vi "Anritsu VNA Read Measurement.vi"(4 "Trace":i8=1 min=1 max=99 step=1, 6 "Channel":i8=1 min=1 max=99 step=1, 7 "Anritsu VNA":T1, 8 "error in (no error)":errorcluster, 11 "VISA Resource Name":refnum<visa-resource-name>) -> (0 "error out":errorcluster, 1 "Parameter":T2={"Stimulus Port"=1, "Response Port"=1} {"Stimulus Port" min=1 step=1; "Response Port" min=1 step=1}, 3 "dup VISA Resource Name":refnum<visa-resource-name>)   [LabVIEW 2011]
doc: "This VI = the HP 8753B is used to read the meausurement format.\n\n0 log magnitude\n1 phase\n2 delay\n3 Smith chart\n4 polar\n5 linear magnitude\n6 standing wave ratio\n7 real\n8 imaginary"
uses:
  tests/S Parameter/TypeDefs/SP Parameter.ctl
  TypeDefs/Anritsu VNA Instrument Info.ctl
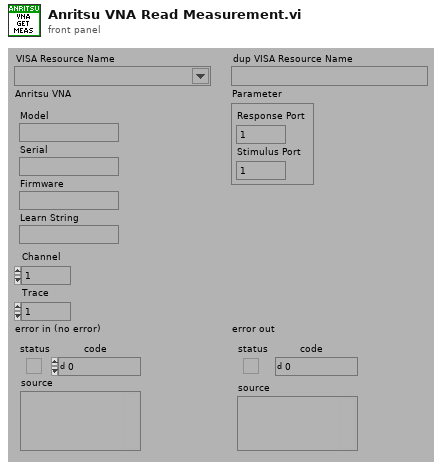
[diagram p1: front panel]
types:
  T1 = typedef "Anritsu VNA Instrument Info.ctl" = cluster{"Model":string, "Serial":string, "Firmware":string, "Learn String":string}
  T2 = typedef "SP Parameter.ctl" = cluster{"Stimulus Port":i8, "Response Port":i8}
  T3 = typedef "Anritsu VNA Model.ctl" = enum16{"Not Supported", "37XXXX", "MS20XXX", "MS462XX", "MS464XX"}
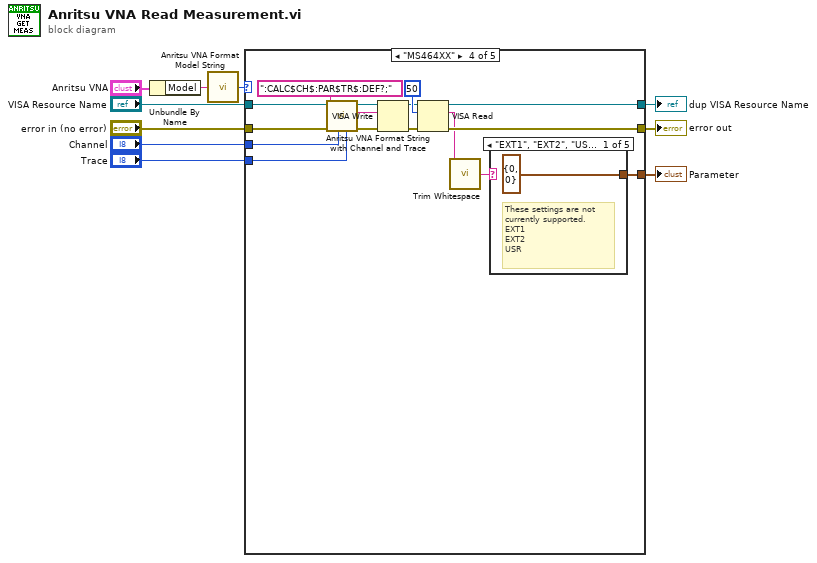
[diagram p0: block diagram]
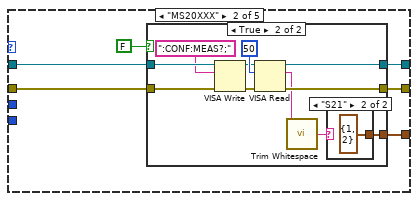
[diagram p3: hidden frame]
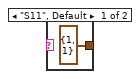
[diagram p5: hidden frame]
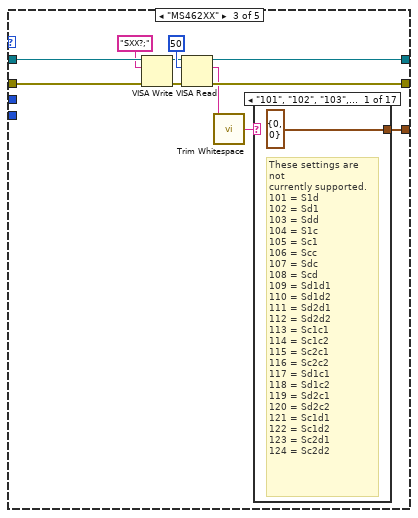
[diagram p6: hidden frame]
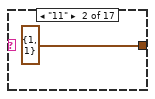
[diagram p7: hidden frame]
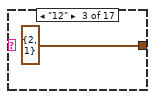
[diagram p8: hidden frame]
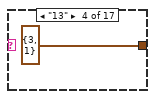
[diagram p9: hidden frame]
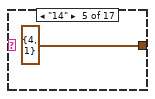
[diagram p10: hidden frame]
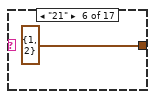
[diagram p11: hidden frame]
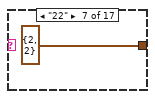
[diagram p12: hidden frame]
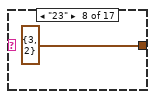
[diagram p13: hidden frame]
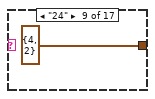
[diagram p14: hidden frame]
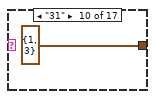
[diagram p15: hidden frame]
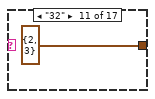
[diagram p16: hidden frame]
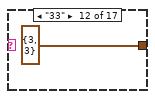
[diagram p17: hidden frame]
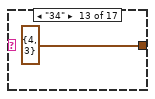
[diagram p18: hidden frame]
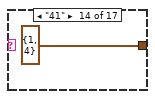
[diagram p19: hidden frame]
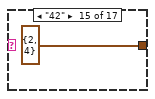
[diagram p20: hidden frame]
diagram:
  n1 = Unbundle By Name("Anritsu VNA") -> ("Model"=w4:string)
  n2 = call "Anritsu VNA Format Model String.vi"("Model"=w4) -> ("Model"=w3:T3)
  n3 = case shown="\"MS464XX\"" w3 {
    tunnel: "VISA Resource Name" -> [w11 w15 w41 w72 w88]
    tunnel: "error in (no error)" -> [w12 w18 w44 w75 w91]
    tunnel: [w12 w17 w43 w74 w90] -> w8
    tunnel: [_ w14 w40 w71 w87] -> w7
    tunnel: [w11 w16 w42 w73 w89] -> w6
    tunnel: "Channel" -> [_ _ _ w63 _]
    tunnel: "Trace" -> [_ _ _ w62 _]
    frame "Not Supported" {
    }
    frame "MS20XXX" {
      n4 = case shown="True" FALSE {
        tunnel: w18 -> [w19 w29]
        tunnel: [w19 w27] -> w17
        tunnel: [w20 w26] -> w16
        tunnel: w15 -> [w20 w25]
        tunnel: [_ w22] -> w14
        frame False {
        }
        frame True {
          n5 = VISA Write(VISA resource name=w25, write buffer=":CONF:MEAS?;", error in (no error)=w29) -> (VISA resource name out=w30:refnum<visa-resource-name>, error out=w28:errorcluster)  [unwired: 1 out]
          n6 = VISA Read(VISA resource name=w30, byte count=u32 50, error in (no error)=w28) -> (VISA resource name out=w26:refnum<visa-resource-name>, read buffer=w24:string, error out=w27:errorcluster)  [unwired: 1 out]
          n7 = call <vilib>:"Trim Whitespace.vi"("string"=w24) -> ("trimmed string"=w23:string)  [unwired: 1 in]
          n8 = case shown="\"S21\"" w23 {
            tunnel: [T2 {"Stimulus Port"=1, "Response Port"=1} ("Display Format") T2 {"Stimulus Port"=1, "Response Port"=2} ("Display Format")] -> w22
            frame "S11", Default {
            }
            frame "S21" {
            }
          }
        }
      }
    }
    frame "MS462XX" {
      n9 = VISA Write(VISA resource name=w41, write buffer="SXX?;", error in (no error)=w44) -> (VISA resource name out=w38:refnum<visa-resource-name>, error out=w37:errorcluster)  [unwired: 1 out]
      n10 = VISA Read(VISA resource name=w38, byte count=u32 50, error in (no error)=w37) -> (VISA resource name out=w42:refnum<visa-resource-name>, read buffer=w36:string, error out=w43:errorcluster)  [unwired: 1 out]
      n11 = call <vilib>:"Trim Whitespace.vi"("string"=w36) -> ("trimmed string"=w35:string)  [unwired: 1 in]
      n12 = case shown="\"101\", \"102\", \"103\", \"104\", \"105\", \"106\", \"107\", \"108\", \"109\", \"110\", \"111\", \"112\", \"113\", \"114\", \"115\", \"116\", \"117\", \"118\", \"119\", \"120\", \"121\", \"122\", \"123\", \"124\", Default" w35 {
        tunnel: [T2 {"Stimulus Port"=0, "Response Port"=0} ("Display Format") T2 {"Stimulus Port"=1, "Response Port"=1} ("Display Format") T2 {"Stimulus Port"=2, "Response Port"=1} ("Display Format") T2 {"Stimulus Port"=3, "Response Port"=1} ("Display Format") T2 {"Stimulus Port"=4, "Response Port"=1} ("Display Format") T2 {"Stimulus Port"=1, "Response Port"=2} ("Display Format") T2 {"Stimulus Port"=2, "Response Port"=2} ("Display Format") T2 {"Stimulus Port"=3, "Response Port"=2} ("Display Format") T2 {"Stimulus Port"=4, "Response Port"=2} ("Display Format") T2 {"Stimulus Port"=1, "Response Port"=3} ("Display Format") T2 {"Stimulus Port"=2, "Response Port"=3} ("Display Format") T2 {"Stimulus Port"=3, "Response Port"=3} ("Display Format") T2 {"Stimulus Port"=4, "Response Port"=3} ("Display Format") T2 {"Stimulus Port"=1, "Response Port"=4} ("Display Format") T2 {"Stimulus Port"=2, "Response Port"=4} ("Display Format") T2 {"Stimulus Port"=3, "Response Port"=4} ("Display Format") T2 {"Stimulus Port"=4, "Response Port"=4} ("Display Format")] -> w40
        frame "101", "102", "103", "104", "105", "106", "107", "108", "109", "110", "111", "112", "113", "114", "115", "116", "117", "118", "119", "120", "121", "122", "123", "124", Default {
          # "These settings are not\ncurrently supported.\n101 = S1d\n102 = Sd1\n103 = Sdd\n104 = S1c\n105 = Sc1\n106 = Scc\n107 = Sdc\n108 = Scd\n109 = Sd1d1\n110 = Sd1d2\n111 = Sd2d1\n112 = Sd2d2\n113 = Sc1c1\n114 = Sc1c2\n115 = Sc2c1\n116 = Sc2c2\n117 = Sd1c1\n118 = Sd1c2\n119 = Sd2c1\n120 = Sd2c2\n121 = Sc1d1\n122 = Sc1d2\n123 = Sc2d1\n124 = Sc2d2"
        }
        frame "11" {
        }
        frame "12" {
        }
        frame "13" {
        }
        frame "14" {
        }
        frame "21" {
        }
        frame "22" {
        }
        frame "23" {
        }
        frame "24" {
        }
        frame "31" {
        }
        frame "32" {
        }
        frame "33" {
        }
        frame "34" {
        }
        frame "41" {
        }
        frame "42" {
        }
        frame "43" {
        }
        frame "44" {
        }
      }
    }
    frame "MS464XX" {
      n13 = call "Anritsu VNA Format String with Channel and Trace.vi"("Trace"=w62, "Channel"=w63, "String"=":CALC$CH$:PAR$TR$:DEF?;") -> ("String Out"=w65:string)  [unwired: 6 out]
      n14 = VISA Write(VISA resource name=w72, write buffer=w65, error in (no error)=w75) -> (VISA resource name out=w69:refnum<visa-resource-name>, error out=w68:errorcluster)  [unwired: 1 out]
      n15 = VISA Read(VISA resource name=w69, byte count=u32 50, error in (no error)=w68) -> (VISA resource name out=w73:refnum<visa-resource-name>, read buffer=w67:string, error out=w74:errorcluster)  [unwired: 1 out]
      n16 = call <vilib>:"Trim Whitespace.vi"("string"=w67) -> ("trimmed string"=w66:string)  [unwired: 1 in]
      n17 = case shown="\"EXT1\", \"EXT2\", \"USR\", Default" w66 {
        tunnel: [T2 {"Stimulus Port"=0, "Response Port"=0} ("Display Format") T2 {"Stimulus Port"=1, "Response Port"=1} ("Display Format") T2 {"Stimulus Port"=1, "Response Port"=2} ("Display Format") T2 {"Stimulus Port"=2, "Response Port"=1} ("Display Format") T2 {"Stimulus Port"=2, "Response Port"=2} ("Display Format")] -> w71
        frame "EXT1", "EXT2", "USR", Default {
          # "These settings are not\ncurrently supported.\nEXT1\nEXT2\nUSR"
        }
        frame "S11" {
        }
        frame "S21" {
        }
        frame "S12" {
        }
        frame "S22" {
        }
      }
    }
    frame "37XXXX" {
      n18 = VISA Write(VISA resource name=w88, write buffer="SXX?;", error in (no error)=w91) -> (VISA resource name out=w85:refnum<visa-resource-name>, error out=w84:errorcluster)  [unwired: 1 out]
      n19 = VISA Read(VISA resource name=w85, byte count=u32 50, error in (no error)=w84) -> (VISA resource name out=w89:refnum<visa-resource-name>, read buffer=w83:string, error out=w90:errorcluster)  [unwired: 1 out]
      n20 = call <vilib>:"Trim Whitespace.vi"("string"=w83) -> ("trimmed string"=w82:string)  [unwired: 1 in]
      n21 = case shown="\"11\", Default" w82 {
        tunnel: [T2 {"Stimulus Port"=1, "Response Port"=1} ("Display Format") T2 {"Stimulus Port"=2, "Response Port"=1} ("Display Format") T2 {"Stimulus Port"=1, "Response Port"=2} ("Display Format") T2 {"Stimulus Port"=2, "Response Port"=2} ("Display Format")] -> w87
        frame "11", Default {
        }
        frame "12" {
        }
        frame "21" {
        }
        frame "22" {
        }
      }
    }
  }
  "Parameter" <- w7
  "dup VISA Resource Name" <- w6
  "error out" <- w8
